vi "Main.vi"() -> ()   [LabVIEW 2020]
doc: "This software acquires data from a simulated source, displays it and performs analysis of the data."
uses:
  Controls/File Type.ctl
  Controls/State.ctl
  Controls/Data.ctl
  Controls/Configuration Settings.ctl
panel:
  in  "File Type":T1
  in  "Open File Location":bool
  in  "Open":bool
  in  "Save":bool
  out "Current State":string
  out "Data":dbl[](graph)
  in  "Reset Settings":bool
  in  "Clear Graph":bool
  in  "Analyze Data":bool
  in  "Acquire Data":bool
  in  "Configure Data":bool
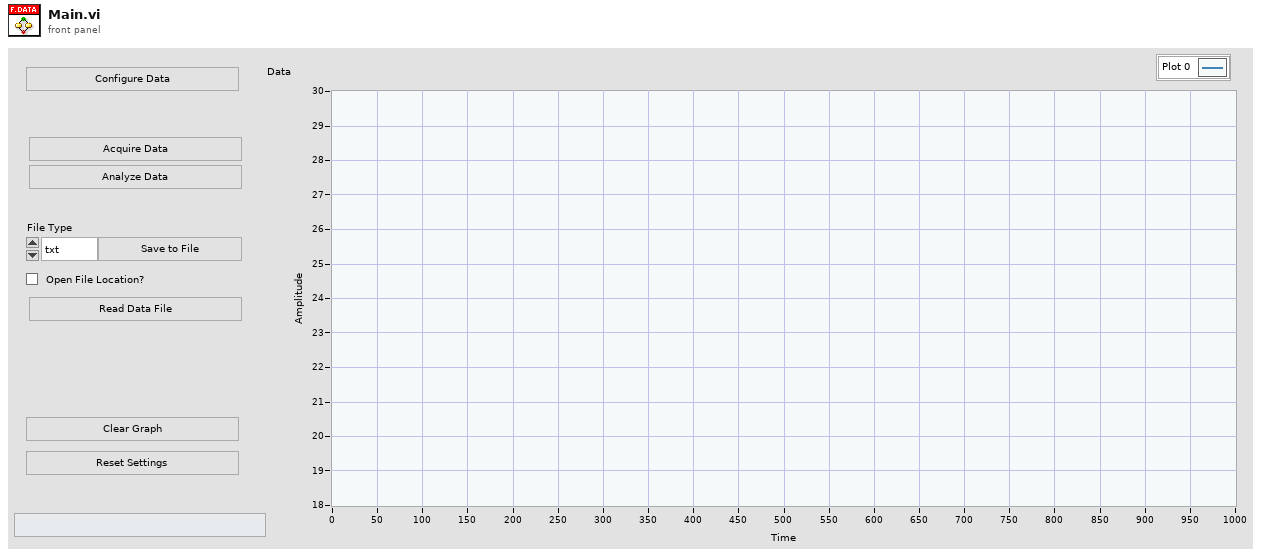
[diagram p1: front panel]
types:
  T1 = typedef "File Type.ctl" = enum16{"txt", "csv", "tdms"}
  T2 = typedef "Data.ctl" = cluster{"Configuration Settings":T3, "Data":dbl[]}
  T3 = typedef "Configuration Settings.ctl" = cluster{"Offset":dbl, "Signal Type":enum16{"Sine Wave", "Triangle Wave", "Square Wave", "Sawtooth Wave"}, "Frequency":dbl, "Amplitude":dbl, "Phase":dbl, "Noise Amplitude":dbl}
  T4 = typedef "State.ctl" = enum16{"Initialize", "Wait for Event", "Configure", "Acquire Data", "Update User Interface", "Reset Data", "Open Data File", "Save Data File", "Clear Data", "Analyse Data", "Stop", "Error"}
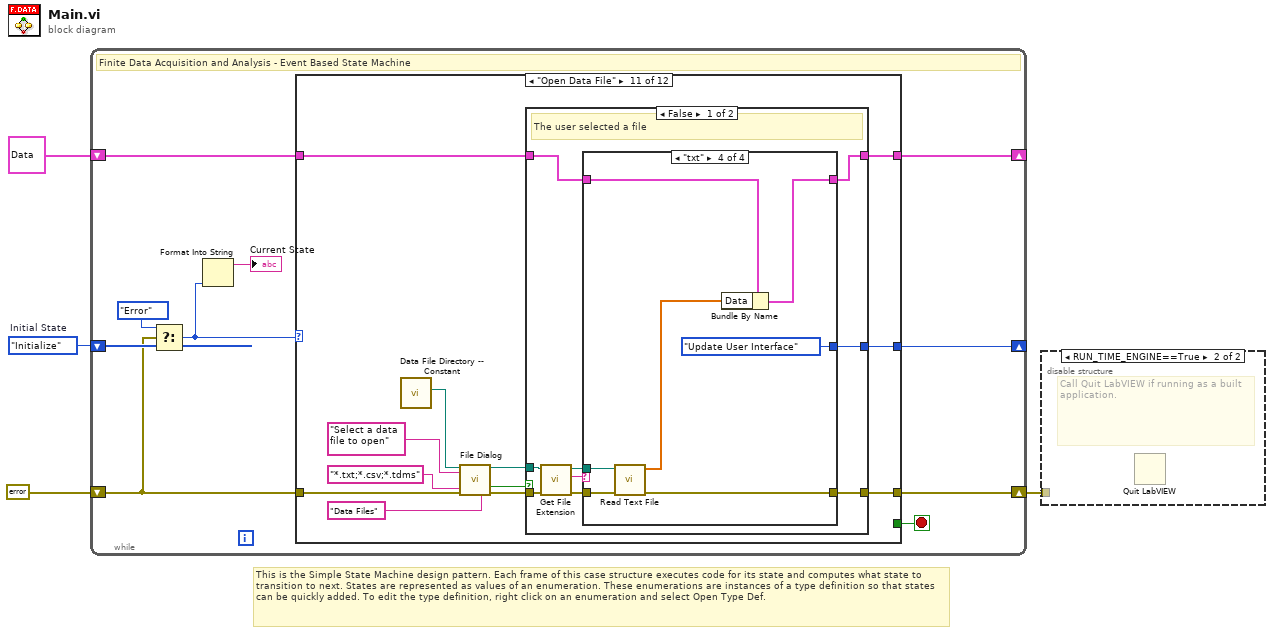
[diagram p0: block diagram]
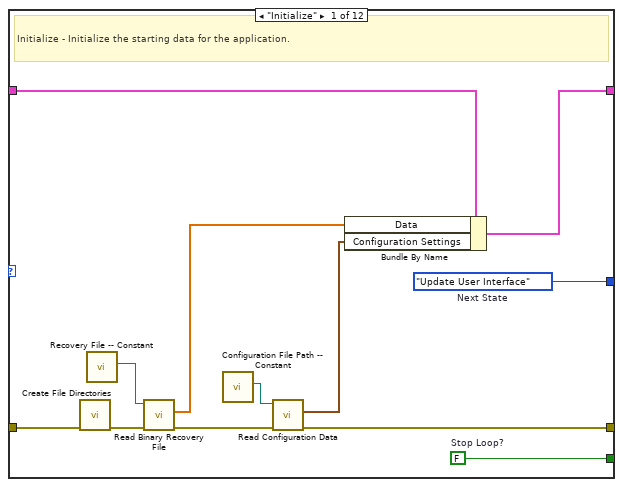
[diagram p2: hidden frame]
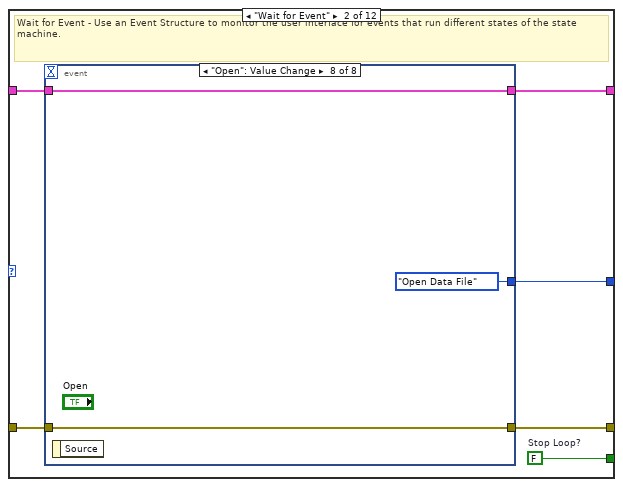
[diagram p3: hidden frame]
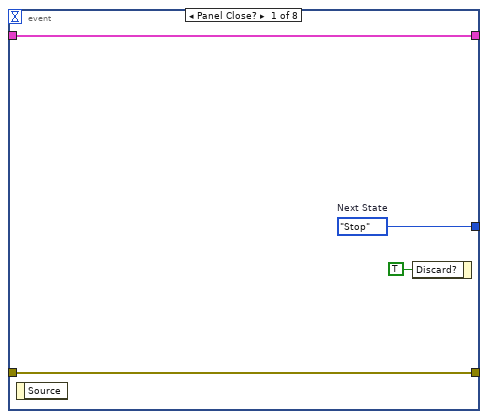
[diagram p4: hidden frame]
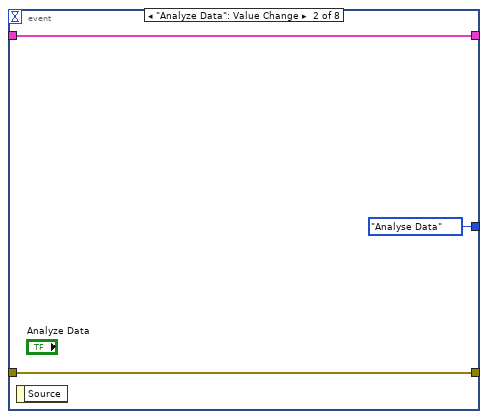
[diagram p5: hidden frame]
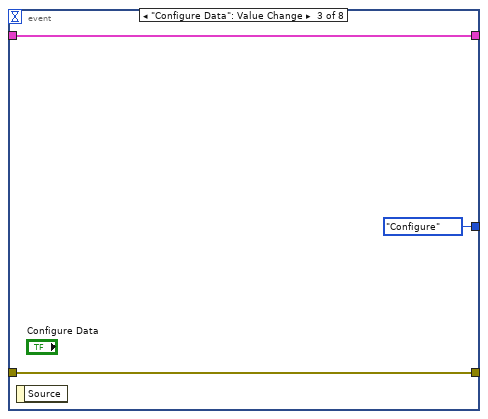
[diagram p6: hidden frame]
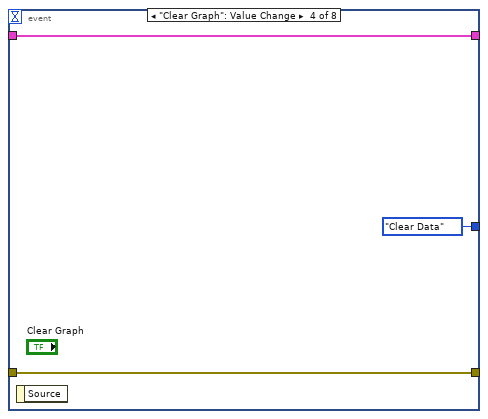
[diagram p7: hidden frame]
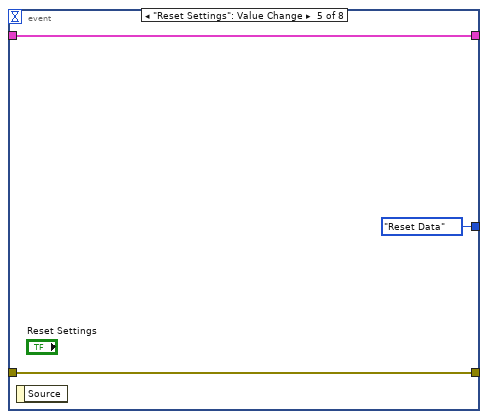
[diagram p8: hidden frame]
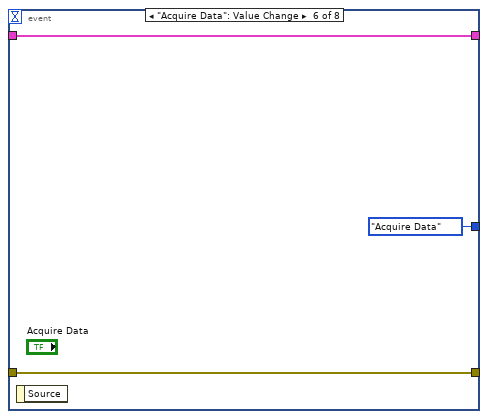
[diagram p9: hidden frame]
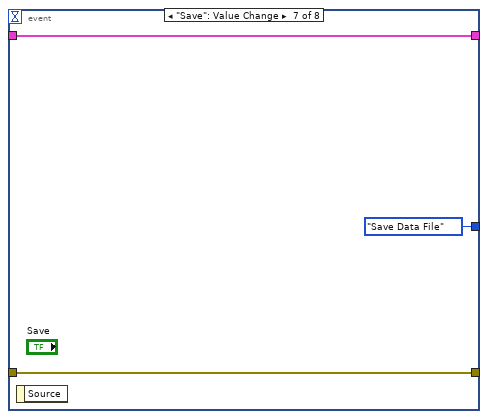
[diagram p10: hidden frame]
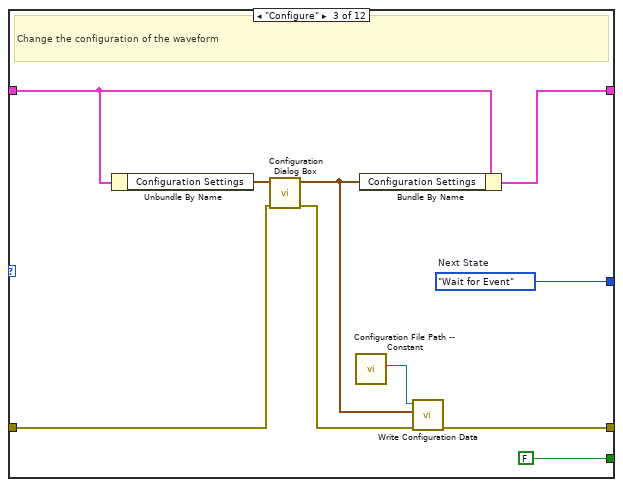
[diagram p11: hidden frame]
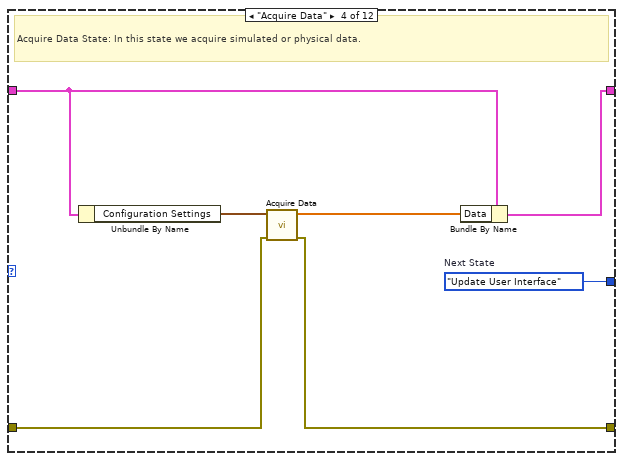
[diagram p12: hidden frame]
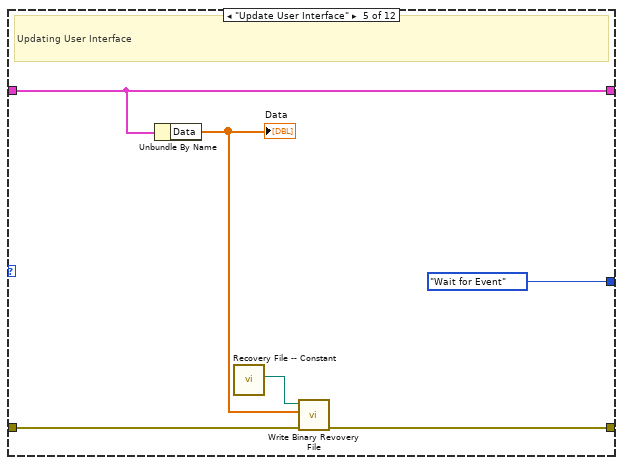
[diagram p13: hidden frame]
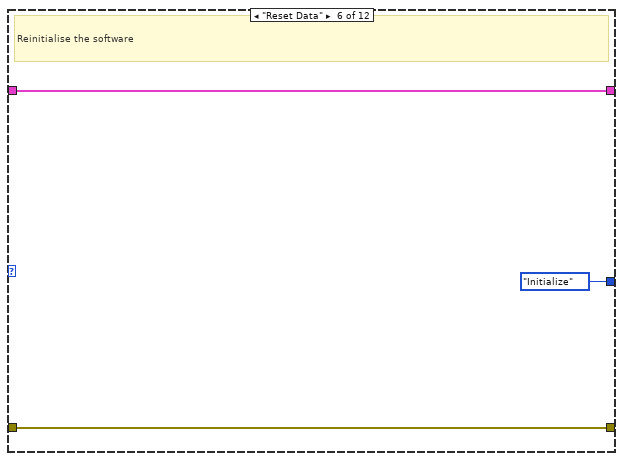
[diagram p14: hidden frame]
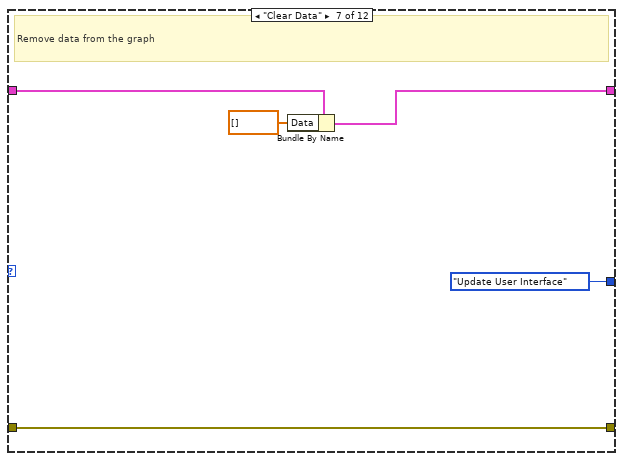
[diagram p15: hidden frame]
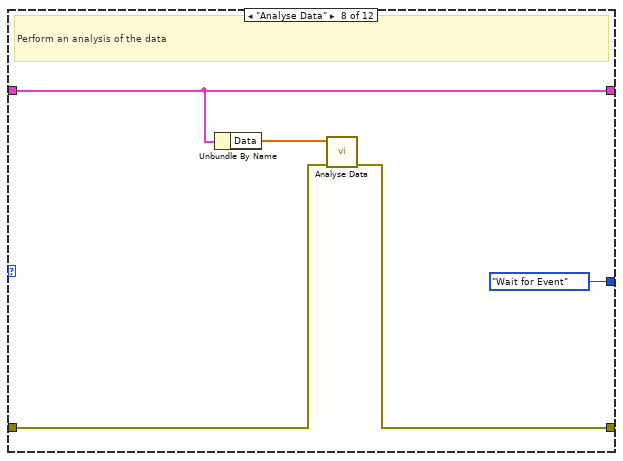
[diagram p16: hidden frame]
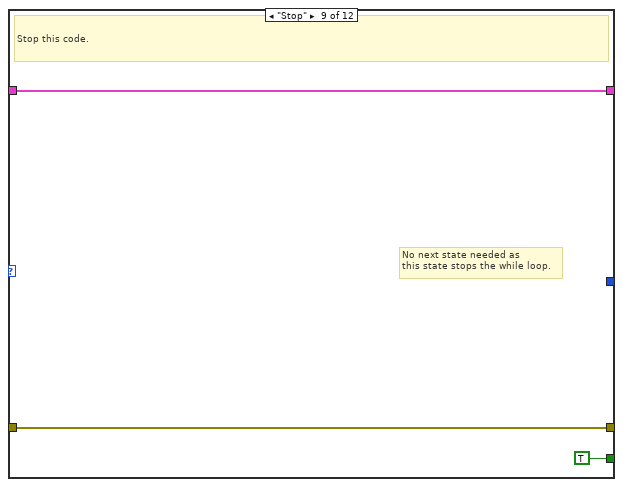
[diagram p17: hidden frame]
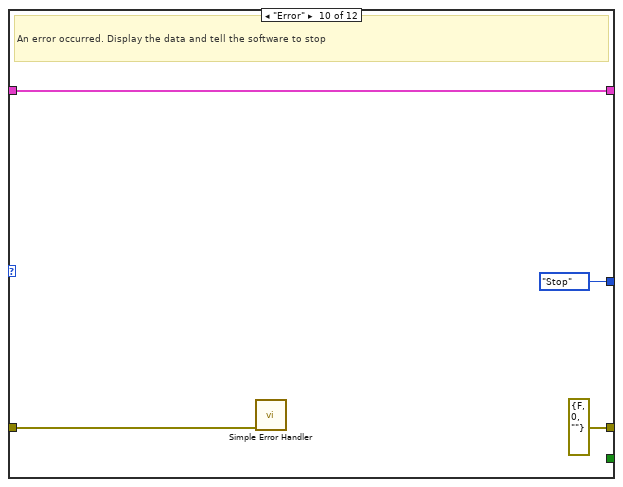
[diagram p18: hidden frame]
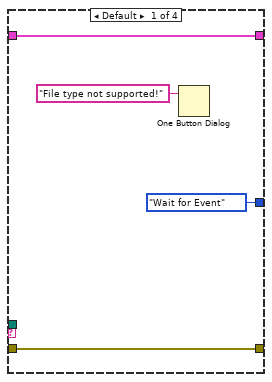
[diagram p19: hidden frame]
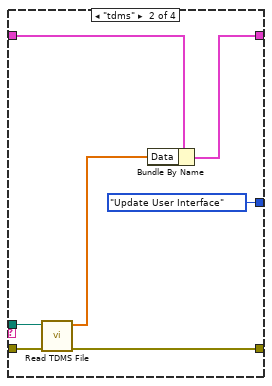
[diagram p20: hidden frame]
diagram:
  w4 = State."Initialize"  # Initial State
  # "This is the Simple State Machine design pattern. Each frame of this case structure executes code for its state and computes what state to transition to next. States are represented as values of an enumeration. These enumerations are instances of a type definition so that states can be quickly added. To edit the type definition, right click on an enumeration and select Open Type Def."
  n1 = while {
    shift-right: [w14] -> _
    shift-left: w4 -> [w9]
    shift-right: [w12] -> _
    shift-left: T2 {"Configuration Settings"={"Offset"=0.0, "Signal Type"=enum."Sine Wave", "Frequency"=10.0, "Amplitude"=1.0, "Phase"=0.0, "Noise Amplitude"=1.0}, "Data"=[]} ("Data") -> [w13]
    shift-right: [w11] -> w1
    shift-left: errorcluster {"status"=FALSE, "code"=0, "source"=""} ("error constant") -> [w10]
    stop <- w5 stop-if-true
    # "Finite Data Acquisition and Analysis - Event Based State Machine"
    n2 = Select(t=State."Error", s=w10, f=w9) -> (s? t:f=w7:T4)
    n3 = Format Into String(w7) -> (resulting string=→"Current State":string)  [unwired: 3 in, 1 out]
    n4 = case shown="\"Open Data File\"" w7 {
      tunnel: [w26 w32 w67 w74 State."Wait for Event" ("(Value Not Used)") State."Initialize" ("(Value Not Used)") State."Update User Interface" ("(Value Not Used)") State."Wait for Event" ("(Value Not Used)") _ State."Stop" ("(Value Not Used)") w106 State."Wait for Event" ("(Value Not Used)")] -> w14
      tunnel: [w25 w31 FALSE ("Stop Loop?") _ _ _ _ _ TRUE ("Stop Loop?") _ _ _] -> w5
      tunnel: w13 -> [w24 w30 w63 w70 w79 w83 w88 w90 w96 w100 w105 w156]
      tunnel: [w23 w29 w62 w68 w79 w83 w85 w90 w96 w100 w104 w156] -> w12
      tunnel: w10 -> [w19 w28 w65 w73 w77 w82 w87 w92 w95 w98 w112 w152]
      tunnel: [w22 w27 w59 w72 w76 w82 w87 w91 w95 errorcluster {"status"=FALSE, "code"=0, "source"=""} ("error constant") w107 w151] -> w11
      frame "Initialize" {
        w25 = FALSE  # Stop Loop?
        w26 = State."Update User Interface"  # Next State
        # "Initialize - Initialize the starting data for the application."
        n5 = call "Create File Directories.vi"("error in (no error)"=w19) -> ("error out"=w16:errorcluster)  [unwired: 10 in]
        n6 = call "Recovery File -- Constant.vi"() -> ("Recovery File Path"=w15:path)  [unwired: 11 in]
        n7 = call "Read Binary Recovery File.vi"("error in (no error)"=w16, "Path"=w15) -> ("error out"=w17:errorcluster, "Data Out"=w18:dbl[])  [unwired: 8 in]
        n8 = call "Configuration File Path -- Constant.vi"() -> ("Configuration File Path"=w20:path)  [unwired: 11 in]
        n9 = call "Read Configuration Data.vi"("error in (no error)"=w17, "Path"=w20) -> ("error out"=w22:errorcluster, "Configuration Settings"=w21:T3)  [unwired: 8 in]
        n10 = Bundle By Name(cluster=w24, "Data"=w18, "Configuration Settings"=w21) -> (w23:T2)
      }
      frame "Wait for Event" {
        w31 = FALSE  # Stop Loop?
        # "Wait for Event - Use an Event Structure to monitor the user interface for events that run different states of the state machine."
        n11 = event shown="[7] \"Open\": Value Change" {
          selector: _ -> [_ _ _ _ _ _ _ _]
          dyn-events: _ -> [_ _ _ _ _ _ _ _]
          timeout: _ -> [_ _ _ _ _ _ _ _]
          tunnel: [w36 State."Analyse Data" ("Next State") State."Configure" ("Next State") State."Clear Data" ("Next State") State."Reset Data" ("Next State") State."Acquire Data" ("Next State") State."Save Data File" ("Next State") State."Open Data File" ("Next State")] -> w32
          tunnel: w30 -> [w35 w39 w42 w45 w48 w51 w54 w57]
          tunnel: [w35 w39 w42 w45 w48 w51 w54 w57] -> w29
          tunnel: w28 -> [w34 w38 w41 w44 w47 w50 w53 w56]
          tunnel: [w34 w38 w41 w44 w47 w50 w53 w56] -> w27
          event Panel Close? {
            w36 = State."Stop"  # Next State
            n12 = event-data() -> ()  [unwired: 1 in, 1 out]
            n13 = event-data("Discard?"=TRUE) -> ()  [unwired: 1 in, 1 out]
          }
          event "Analyze Data": Value Change {
            n14 = event-data() -> ()  [unwired: 1 in, 1 out]
          }
          event "Configure Data": Value Change {
            n15 = event-data() -> ()  [unwired: 1 in, 1 out]
          }
          event "Clear Graph": Value Change {
            n16 = event-data() -> ()  [unwired: 1 in, 1 out]
          }
          event "Reset Settings": Value Change {
            n17 = event-data() -> ()  [unwired: 1 in, 1 out]
          }
          event "Acquire Data": Value Change {
            n18 = event-data() -> ()  [unwired: 1 in, 1 out]
          }
          event "Save": Value Change {
            n19 = event-data() -> ()  [unwired: 1 in, 1 out]
          }
          event "Open": Value Change {
            n20 = event-data() -> ()  [unwired: 1 in, 1 out]
          }
        }
      }
      frame "Configure" {
        w67 = State."Wait for Event"  # Next State
        # "Change the configuration of the waveform"
        n21 = Unbundle By Name(w63) -> ("Configuration Settings"=w64:T3)
        n22 = call "Configuration Dialog Box.vi"("error in (no error)"=w65, "Configuration Settings In"=w64) -> ("error out"=w60:errorcluster, "Configuration Settings Out"=w61:T3)  [unwired: 8 in]
        n23 = call "Configuration File Path -- Constant.vi"() -> ("Configuration File Path"=w58:path)  [unwired: 11 in]
        n24 = Bundle By Name(cluster=w63, "Configuration Settings"=w61) -> (w62:T2)
        n25 = call "Write Configuration Data.vi"("error in (no error)"=w60, "Configuration Settings"=w61, "Path"=w58) -> ("error out"=w59:errorcluster)  [unwired: 8 in]
      }
      frame "Acquire Data" {
        w74 = State."Update User Interface"  # Next State
        # "Acquire Data State: In this state we acquire simulated or physical data."
        n26 = Unbundle By Name(w70) -> ("Configuration Settings"=w71:T3)
        n27 = call "Acquire Data.vi"("error in (no error)"=w73, "Configuration Settings"=w71) -> ("error out"=w72:errorcluster, "Data Out"=w69:dbl[])  [unwired: 8 in]
        n28 = Bundle By Name(cluster=w70, "Data"=w69) -> (w68:T2)
      }
      frame "Update User Interface" {
        # "Updating User Interface"
        n29 = Unbundle By Name(w79) -> ("Data"=w78:dbl[])
        "Data" <- w78
        n30 = call "Recovery File -- Constant.vi"() -> ("Recovery File Path"=w75:path)  [unwired: 11 in]
        n31 = call "Write Binary Revovery File.vi"("error in (no error)"=w77, "Data In"=w78, "Path"=w75) -> ("error out"=w76:errorcluster)  [unwired: 8 in]
      }
      frame "Reset Data" {
        # "Reinitialise the software"
      }
      frame "Clear Data" {
        # "Remove data from the graph"
        n32 = Bundle By Name(cluster=w88, "Data"=dbl[] []) -> (w85:T2)
      }
      frame "Analyse Data" {
        # "Perform an analysis of the data"
        n33 = Unbundle By Name(w90) -> ("Data"=w89:dbl[])
        n34 = call "Analyse Data.vi"("error in (no error)"=w92, "Data In"=w89) -> ("error out"=w91:errorcluster)  [unwired: 9 in]
      }
      frame "Stop" {
        # "No next state needed as \nthis state stops the while loop."
        # "Stop this code."
      }
      frame "Error" {
        # "An error occurred. Display the data and tell the software to stop"
        n35 = call <vilib>:"Simple Error Handler.vi"("error in (no error)"=w98) -> ()  [unwired: 4 in, 5 out]
      }
      frame "Open Data File" {
        n36 = call "Data File Directory -- Constant.vi"() -> ("Data File Directory"=w101:path)  [unwired: 11 in]
        n37 = call "File Dialog"("start path"=w101, "prompt"="Select a data file to open", "error in"=w112, "pattern (all files)"="*.txt;*.csv;*.tdms", "pattern label"="Data Files") -> ("selected path"=w103:path, "cancelled"=w108:bool, "error out"=w102:errorcluster)  [unwired: 7 in, 1 out]
        n38 = case shown="False" w108 {
          tunnel: [w118 w149] -> w107
          tunnel: [w119 State."Wait for Event" ("t")] -> w106
          tunnel: w105 -> [w121 w147]
          tunnel: [w120 w147] -> w104
          tunnel: w103 -> [w116 _]
          tunnel: w102 -> [w115 _]
          frame False {
            # "The user selected a file"
            n39 = call <vilib>:"Get File Extension.vi"("error in (no error)"=w115, "file"=w116) -> ("error out"=w117:errorcluster, "lowercase file extension"=w114:string, "dup file"=w113:path)  [unwired: 5 in, 2 out]
            n40 = case shown="\"txt\"" w114 {
              tunnel: w121 -> [w125 w132 w139 w146]
              tunnel: [w125 w131 w138 w145] -> w120
              tunnel: [State."Wait for Event" ("t") State."Update User Interface" ("t") State."Update User Interface" ("t") State."Update User Interface" ("t")] -> w119
              tunnel: [w122 w127 w133 w141] -> w118
              tunnel: w117 -> [w122 w128 w135 w142]
              tunnel: w113 -> [_ w129 w136 w143]
              frame Default {
                n41 = One Button Dialog(message="File type not supported!") -> ()  [unwired: 1 in, 1 out]
              }
              frame "tdms" {
                n42 = call "Read TDMS File.vi"("error in (no error)"=w128, "Path"=w129) -> ("error out"=w127:errorcluster, "Data"=w126:dbl[])  [unwired: 8 in]
                n43 = Bundle By Name(cluster=w132, "Data"=w126) -> (w131:T2)
              }
              frame "csv" {
                n44 = call "Read CSV File.vi"("error in (no error)"=w135, "Path"=w136) -> ("error out"=w133:errorcluster, "Data"=w134:dbl[])  [unwired: 8 in]
                n45 = Bundle By Name(cluster=w139, "Data"=w134) -> (w138:T2)
              }
              frame "txt" {
                n46 = call "Read Text File.vi"("error in (no error)"=w142, "Path"=w143) -> ("error out"=w141:errorcluster, "Data"=w140:dbl[])  [unwired: 8 in]
                n47 = Bundle By Name(cluster=w146, "Data"=w140) -> (w145:T2)
              }
            }
          }
          frame True {
            # "The user cancelled the file dialog"
            n48 = call <vilib>:"Clear Errors.vi"("specific error code to clear (0: all)"=43) -> ("error out"=w149:errorcluster)  [unwired: 5 in, 1 out]
          }
        }
      }
      frame "Save Data File" {
        n49 = Unbundle By Name(w156) -> ("Data"=w154:dbl[])
        n50 = call "Save Data File.vi"("error in (no error)"=w152, "Open File Location"="Open File Location", "Data"=w154, "File Type"="File Type") -> ("error out"=w151:errorcluster)  [unwired: 7 in]
      }
    }
  }
  n51 = disable-structure shown="RUN_TIME_ENGINE==True" {
    disable-tunnel: w1 -> [_ _]
    frame condition #0 (active) {
    }
    frame condition #1 {
      # "Call Quit LabVIEW if running as a built application."
      n52 = Quit LabVIEW() -> ()  [unwired: 1 in]
    }
  }
